vi "GetDefaultControlType.vi"(8 "Error In":errorcluster) -> (0 "Error Out":errorcluster, 2 "Default control style valid?":bool, 3 "Error control type":T1)   [LabVIEW 2017, in "ErrorStructureDrawer.lvlib"]
doc: "Gets the default control type from the LabVIEW INI file."
uses:
  ErrorStructureDrawer.lvlib
  Controls/ErrorControlType.ctl
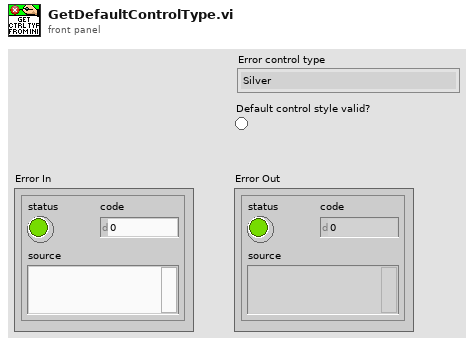
[diagram p1: front panel]
types:
  T1 = typedef "ErrorStructureDrawer.lvlib/ErrorControlType.ctl" = enum16{"Silver", "Modern", "Classic", "LabVIEW default", "NXG"}
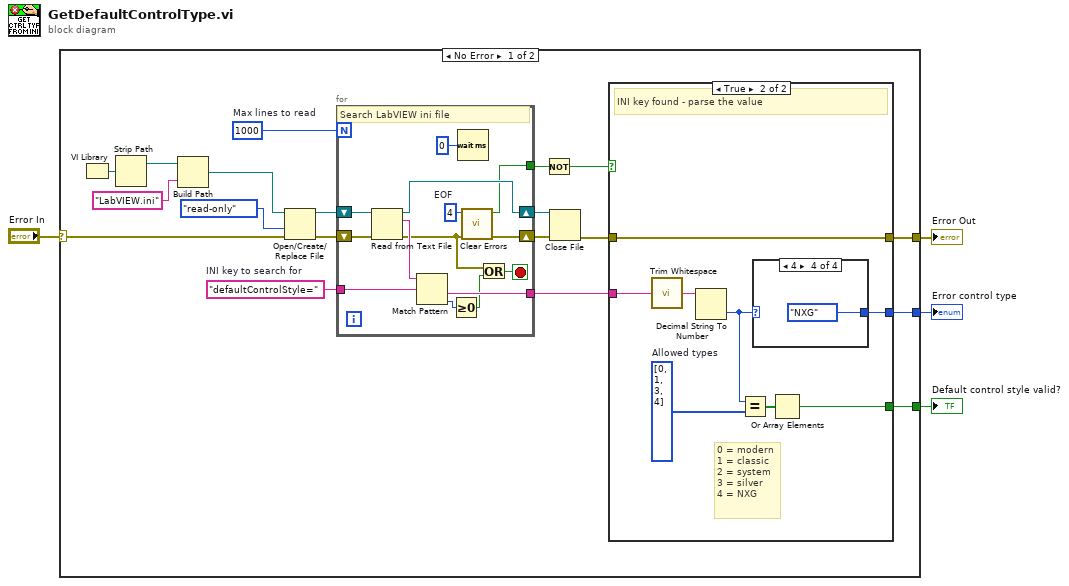
[diagram p0: block diagram]
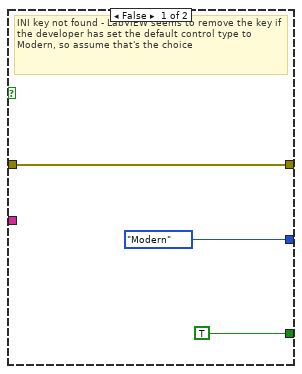
[diagram p2: hidden frame]
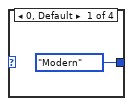
[diagram p3: hidden frame]
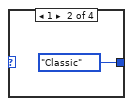
[diagram p4: hidden frame]
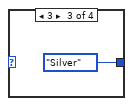
[diagram p5: hidden frame]
diagram:
  n1 = case shown="No Error" "Error In" {
    selector: "Error In" -> [w9 w53]
    tunnel: [w7 _] -> w4
    tunnel: [w10 _] -> w3
    tunnel: [w6 w53] -> w1
    frame No Error {
      w13 = "defaultControlStyle="  # INI key to search for
      w14 = 1000  # Max lines to read
      n2 = VI Library() -> (path=w23:path)
      n3 = Strip Path(path=w23) -> (stripped path=w22:path)  [unwired: 1 out]
      n4 = Build Path(base path=w22, name or relative path="LabVIEW.ini") -> (appended path=w20:path)
      n5 = Open/Create/Replace File(file path (use dialog)=w20, error in=w9, access (0:read/write)=enum16{"read/write", "read-only", "write-only"}."read-only") -> (refnum out=w18:refnum<file>, error out=w17:errorcluster)  [unwired: 3 in, 1 out]
      n6 = for {
        N: w14 -> [_]
        shift-right: [w50] -> w15
        shift-left: w18 -> [w52]
        shift-right: [w49] -> w16
        shift-left: w17 -> [w51]
        tunnel: [w48] -> w11
        tunnel: w13 -> [w45]
        tunnel: [w44] -> w12
        stop <- w41 stop-if-true
        w40 = 4  # EOF
        # "Search LabVIEW ini file"
        n7 = Read from Text File(file (use dialog)=w52, error in=w51) -> (refnum out=w50:refnum<file>, text=w46:string, error out=w39:errorcluster)  [unwired: 2 in, 1 out]
        n8 = Match Pattern(string=w46, regular expression=w45) -> (after substring=w44:string, offset past match=w43:i32)  [unwired: 1 in, 2 out]
        n9 = Greater Or Equal To 0?(x=w43) -> (x >= 0?=w42:bool)
        n10 = Wait (ms)(milliseconds to wait=u32 0) -> ()  [unwired: 1 out]
        n11 = call <vilib>:"Clear Errors.vi"("error in (no error)"=w39, "specific error code to clear (0: all)"=w40) -> ("error out"=w49:errorcluster, "specific error cleared?"=w48:bool)  [unwired: 4 in]
        n12 = Or(x=w39, y=w42) -> (x .or. y?=w41:bool)
      }
      n13 = Not(x=w11) -> (.not. x?=w8:bool)
      n14 = Close File(refnum=w15, error in=w16) -> (error out=w5:errorcluster)  [unwired: 1 out]
      n15 = case shown="True" w8 {
        tunnel: w12 -> [_ w34]
        tunnel: [ErrorControlType."Modern" ("Error control type") w32] -> w10
        tunnel: [TRUE w28] -> w7
        tunnel: [w26 w27] -> w6
        tunnel: w5 -> [w26 w27]
        frame False {
          # "INI key not found - LabVIEW seems to remove the key if the developer has set the default control type to Modern, so assume that's the choice"
        }
        frame True {
          w31 = i32[] [0, 1, 3, 4]  # Allowed types
          # "0 = modern\n1 = classic\n2 = system\n3 = silver\n4 = NXG"
          # "INI key found - parse the value"
          n16 = call <vilib>:"Trim Whitespace.vi"("string"=w34) -> ("trimmed string"=w33:string)  [unwired: 1 in]
          n17 = Decimal String To Number(string=w33) -> (number=w30:i32)  [unwired: 2 in, 1 out]
          n18 = Equal?(x=w30, y=w31) -> (x = y?=w29:bool[])
          n19 = case shown="4" w30 {
            tunnel: [ErrorControlType."Modern" ("Error control type") ErrorControlType."Classic" ("Error control type") ErrorControlType."Silver" ("Error control type") ErrorControlType."NXG" ("Error control type")] -> w32
            frame 0, Default {
            }
            frame 1 {
            }
            frame 3 {
            }
            frame 4 {
            }
          }
          n20 = Or Array Elements(Boolean array=w29) -> (logical OR=w28:bool)
        }
      }
    }
    frame Error {
    }
  }
  "Default control style valid?" <- w4
  "Error control type" <- w3
  "Error Out" <- w1
